vi "Get Test Conditions.vi"(0 "Fuel":string(combo), 1 "CSV Array":string[][](array[string]), 3 "indices":T1={"fuel"=0, "oxidizer"=1, "diluent"=2, "diluent_mol_frac"=3, "equivalence"=4, "init_pressure"=5, "p_f"=6, "p_ox"=7, "p_dil"=8}, 5 "Oxidizer":string(combo), 9 "Diluent":string(combo), 11 "Equivalence Ratio":string(combo), 12 "Diluent Mole Fraction":string(combo), 13 "Initial Pressure":string(combo)) -> (4 "Test Found":bool, 6 "Fuel Cutoff Pressure":dbl, 8 "Test row":string[](array[string]), 10 "Oxidizer Cutoff Pressure":dbl, 14 "f_a_st":dbl, 15 "Diluent Cutoff Pressure":dbl)   [LabVIEW 2018]
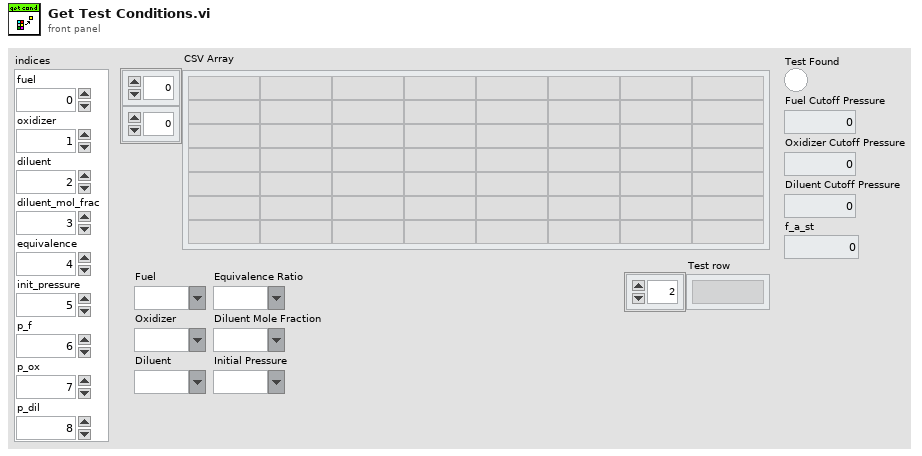
[diagram p1: front panel]
types:
  T1 = cluster{"fuel":i32, "oxidizer":i32, "diluent":i32, "diluent_mol_frac":i32, "equivalence":i32, "init_pressure":i32, "p_f":i32, "p_ox":i32, "p_dil":i32}
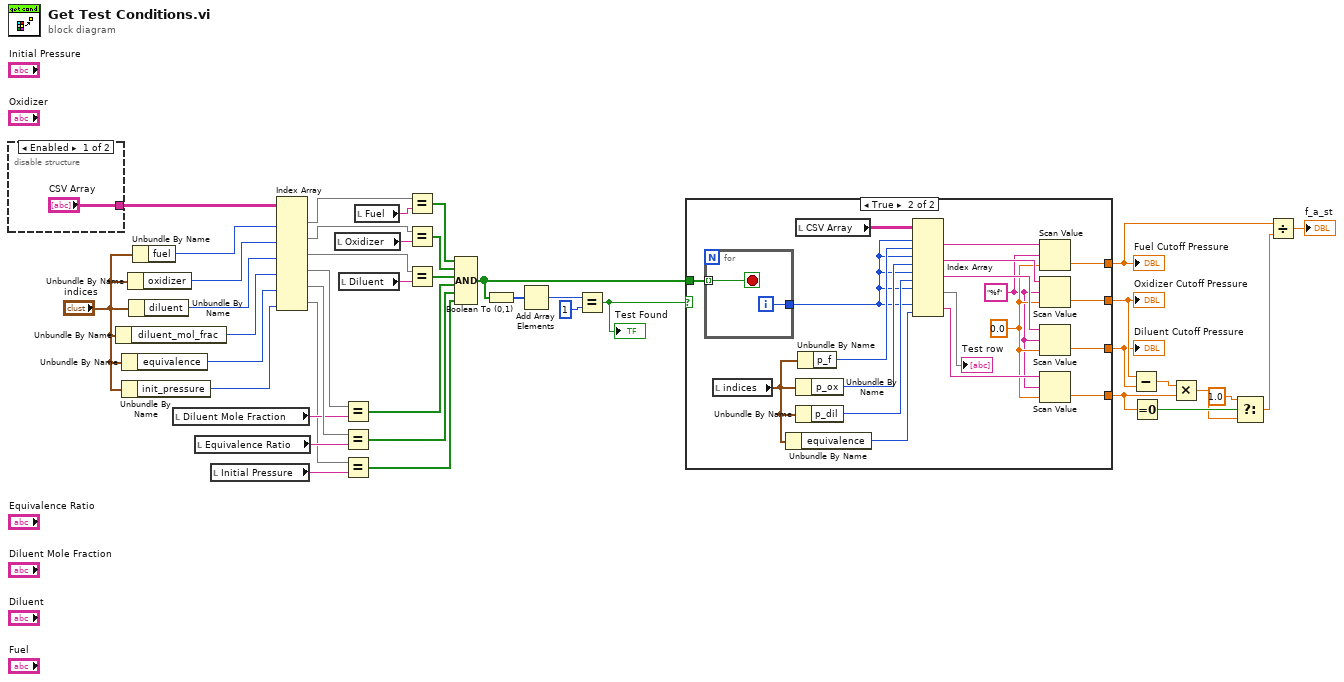
[diagram p0: block diagram]
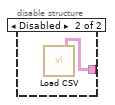
[diagram p2: hidden frame]
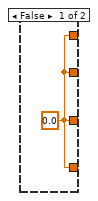
[diagram p3: hidden frame]
diagram:
  n1 = disable-structure shown="Enabled" {
    disable-tunnel: ["CSV Array" w43] -> w12
    frame Enabled {
    }
    frame Disabled {
      n2 = call "Load CSV.vi"() -> ("CSV Array"=w43:string[][])  [unwired: 10 in, 9 out]
    }
  }
  n3 = Unbundle By Name("indices") -> ("diluent_mol_frac"=w33:i32)
  n4 = Unbundle By Name("indices") -> ("equivalence"=w32:i32)
  n5 = Unbundle By Name("indices") -> ("init_pressure"=w16:i32)
  n6 = Unbundle By Name("indices") -> ("oxidizer"=w36:i32)
  n7 = Unbundle By Name("indices") -> ("diluent"=w34:i32)
  n8 = Unbundle By Name("indices") -> ("fuel"=w37:i32)
  n9 = local read "Diluent Mole Fraction"() -> (w23:string)
  n10 = local read "Equivalence Ratio"() -> (w22:string)
  n11 = local read "Initial Pressure"() -> (w14:string)
  n12 = Index Array(array=w12, index (col) #1=w37, index (col) #2=w36, index (col) #3=w34, index (col) #4=w33, index (col) #5=w32, index (col) #6=w16) -> (element #1=w40:string[], element #2=w39:string[], element #3=w30:string[], element #4=w29:string[], element #5=w28:string[], element #6=w15:string[])  [unwired: 6 in]
  n13 = local read "Oxidizer"() -> (w38:string)
  n14 = local read "Diluent"() -> (w24:string)
  n15 = Equal?(x=w29, y=w23) -> (x = y?=w26:bool[])
  n16 = Equal?(x=w28, y=w22) -> (x = y?=w25:bool[])
  n17 = Equal?(x=w15, y=w14) -> (x = y?=w13:bool[])
  n18 = local read "Fuel"() -> (w41:string)
  n19 = Equal?(x=w40, y=w41) -> (x = y?=w35:bool[])
  n20 = Equal?(x=w39, y=w38) -> (x = y?=w31:bool[])
  n21 = Equal?(x=w30, y=w24) -> (x = y?=w27:bool[])
  n22 = Compound Arithmetic op=AND(w35, w31, w27, w26, w25, w13) -> (w17:bool[])
  n23 = Boolean To (0,1)(Boolean=w17) -> (0, 1=w21:i16[])
  n24 = Add Array Elements(numeric array=w21) -> (sum=w20:i16)
  n25 = Equal?(x=w20, y=i16 1) -> (x = y?=w18:bool)
  "Test Found" <- w18
  n26 = case shown="True" w18 {
    tunnel: w17 -> [_ w63]
    tunnel: [w44 w60] -> w3
    tunnel: [w44 w57] -> w9
    tunnel: [w44 w56] -> w8
    tunnel: [w44 w46] -> w6
    frame False {
      w44 = 0.0
    }
    frame True {
      w45 = "%f" ("format string")
      w47 = 0.0
      n27 = for {
        tunnel: w63 -> [w65] mode=indexing
        tunnel: [w64] -> w51
        i -> [w64]
        stop <- w65 stop-if-true
      }
      n28 = local read "indices"() -> (w50:T1)
      n29 = Unbundle By Name(w50) -> ("equivalence"=w49:i32)
      n30 = local read "CSV Array"() -> (w62:string[][])
      n31 = Unbundle By Name(w50) -> ("p_ox"=w54:i32)
      n32 = Unbundle By Name(w50) -> ("p_dil"=w55:i32)
      n33 = Unbundle By Name(w50) -> ("p_f"=w53:i32)
      n34 = Index Array(array=w62, index (row) #1=w51, index (col) #1=w53, index (row) #2=w51, index (col) #2=w54, index (row) #3=w51, index (col) #3=w55, index (row) #4=w51, index (row) #5=w51, index (col) #5=w49) -> (element #1=w61:string, element #2=w58:string, element #3=w59:string, element #4=→"Test row":string[], element #5=w48:string)  [unwired: 1 in]
      n35 = Scan Value(string=w61, format string=w45, default (0 dbl)=w47) -> (value=w60:dbl)  [unwired: 1 out]
      n36 = Scan Value(string=w58, format string=w45, default (0 dbl)=w47) -> (value=w57:dbl)  [unwired: 1 out]
      n37 = Scan Value(string=w59, format string=w45, default (0 dbl)=w47) -> (value=w56:dbl)  [unwired: 1 out]
      n38 = Scan Value(string=w48, format string=w45, default (0 dbl)=w47) -> (value=w46:dbl)  [unwired: 1 out]
    }
  }
  "Diluent Cutoff Pressure" <- w8
  "Fuel Cutoff Pressure" <- w3
  "Oxidizer Cutoff Pressure" <- w9
  n39 = Subtract(x=w9, y=w8) -> (x-y=w7:dbl)
  n40 = Equal To 0?(x=w6) -> (x = 0?=w10:bool)
  n41 = Multiply(x=w7, y=w6) -> (x*y=w5:dbl)
  n42 = Select(t=1.0, s=w10, f=w5) -> (s? t:f=w2:dbl)
  n43 = Divide(x=w3, y=w2) -> (x/y=→"f_a_st":dbl)
